vi "GetRxPower(LC).vi"(0 "SAVE FILE PATH":path=path "C:/RageATE/Automated Tests/Tetra WAM/DVT/rxdata.csv", 1 "CloseCOM4":bool, 2 "RXAnt":i32=1, 3 "RunAM_Init":bool=TRUE, 4 "UseFastData(T)":bool=TRUE, 5 "error in (no error)":errorcluster, 6 "dBFS Ofset":dbl, 7 "SAVE TO FILE(T)":bool, 8 "INPUT FILE PATH":path, 9 "INPUT FROM FILE(T)":bool, 11 "CF(MHZ)":dbl=10.0 min=0.0 max=150.0 format="%#_13g", 13 "BW(MHZ)":dbl=10.0 format="%#_13g", 15 "AMInitDyn(t)":bool, 18 "#ofAvg":i32=1) -> (10 "band (dbfs/mhz)":dbl[](array[numeric])=[-40.41732245857817, 9.96580361504641] format="%#_4g", 12 "peak (dbfs/mhz)":dbl[](array[numeric])=[-43.929, 10.039082] format="%#_8g", 14 "Locked?(T)":bool=TRUE, 16 "Am_Init_Flag":bool, 19 "error out":errorcluster={"status"=FALSE, "code"=1073676418, "source"="VISA Close in GetRxPower.vi"})   [LabVIEW 2018]
uses:
  Tetra_Globals.vi
  Initialize References/Sequence Globals.vi
panel:
  out "PyBase":string
  out "Navg":string
  out "Fs":string
  in  "ForceRevC(t)":bool
  out "vipath":string
  out "antenna":string
  out "match substring":string
  out "py_comport":string
  out "gui working directory":path=path "C:/TetraLabGUI"
  in  "Plot":u16(ring) items=["NoPlot", "Plot"]
  out "standard error":string
  out "UseAVG(t)":bool
  out "cmd_in":string
  out "standard output":string="2939 49c4\r\n403 6001\r\nFound COM4\r\nseq off\r\nwr reg 0x02 0x0400\r\nwr reg 0x03 0x0000\r\nwr reg 0x04 1032\r\nwr reg 0x05 4\r\nwr reg 0x06 10\r\nwr reg 0x08 256\r\nwr reg 0x09 51\r\nwr reg 0x0A 4\r\nwr reg 0x0E 8000\r\nwr reg 0x0F 0x5555\r\nwr reg 0x10 0x0055\r\nwr reg 0x11 0xAAAA\r\nwr reg 0x12 0x00AA\r\nwr reg 0x1A 0x0000\r\nwr reg 0x1B 0x0000\r\nwr reg 0x17 0x0300\r\nwr reg 0x18 0x0000\r\nsos\r\n"
  out "Time(ms)":u32=1465
  out "start":u32=9009331
  out "console  output":string="b'OK\\n\\r'\r\n[-26 -27 -23 ... -15 -16 -17]\r\nMax Value: -43.929 dBFS at 10.039082 MHz\r\nCF_OUT(MHz) = 9.96580361504641\r\nBP_OUT(dBfs) = -40.41732245857817\r\n"
  # "Input Dialog. Check \"Show Plot\" if desired"
  # "7.06"
  # "File Path Dialog. Check if file save desired"
  # "Band  & Peak Power Outputs"
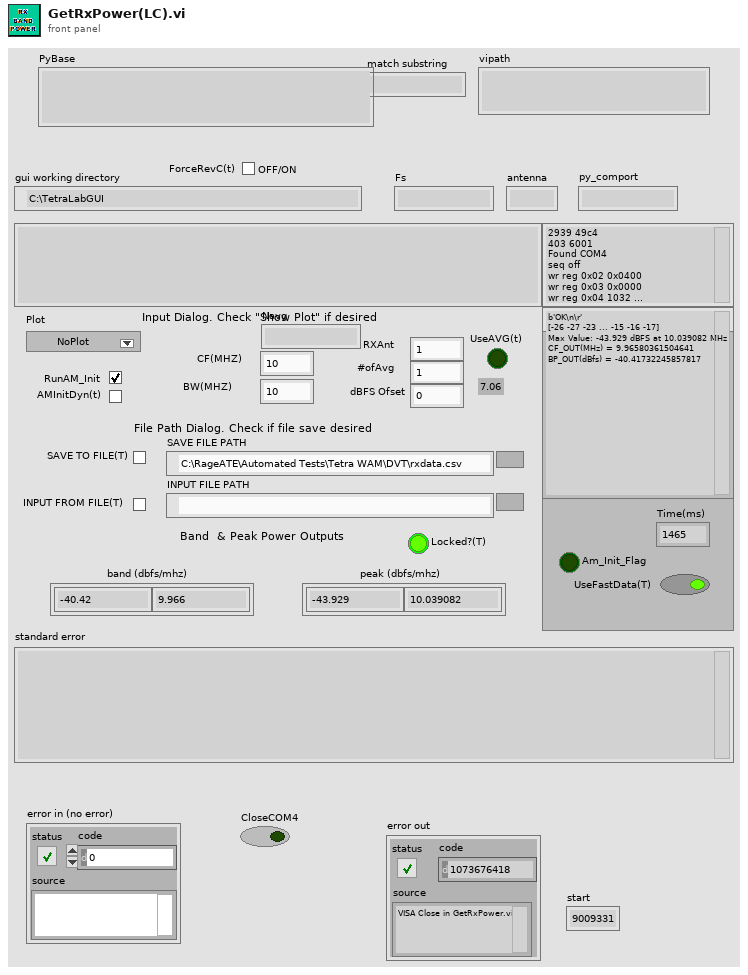
[diagram p1: front panel]
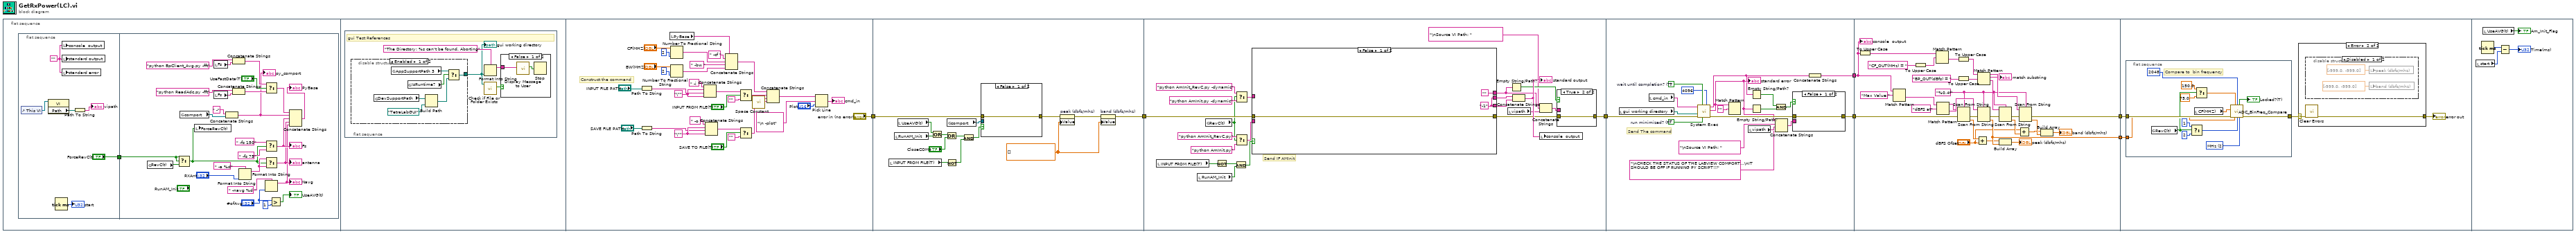
[diagram p0: block diagram]
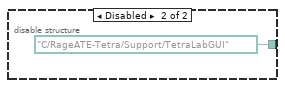
[diagram p2: hidden frame]
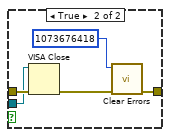
[diagram p4: hidden frame]
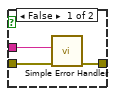
[diagram p5: hidden frame]
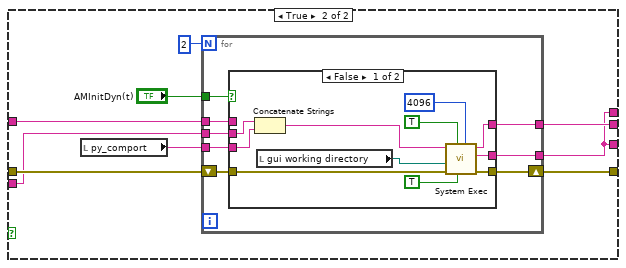
[diagram p6: hidden frame]
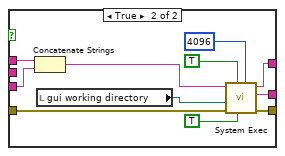
[diagram p7: hidden frame]
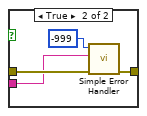
[diagram p8: hidden frame]
diagram:
  n1 = flat-sequence {
    tunnel: ["error in (no error)"] -> w1
    tunnel: [w100] -> w2
    tunnel: w1 -> [w99]
    tunnel: [w119] -> w5
    tunnel: w2 -> [w128]
    tunnel: [w189] -> w7
    tunnel: [w184] -> w6
    tunnel: w5 -> [w191]
    tunnel: w7 -> [w227]
    tunnel: w6 -> [w211]
    tunnel: [w212] -> w4
    tunnel: [w210] -> w3
    tunnel: w4 -> [w233]
    tunnel: w3 -> [w232]
    frame #0 {
      n2 = flat-sequence {
        tunnel: ["ForceRevC(t)"] -> w8
        tunnel: w8 -> [w35]
        frame #0 {
          w13 = ""
          n3 = control-ref of="This VI"() -> (w10:refnum<vi>)
          n4 = property class="VI"(reference=w10) -> ("Path"=w11:path)  [unwired: 1 in, 2 out]
          n5 = Tick Count (ms)() -> (millisecond timer value=→"start":u32)
          n6 = local write "console  output"(w13) -> ()
          n7 = local write "standard output"(w13) -> ()
          n8 = local write "standard error"(w13) -> ()
          n9 = Path To String(path=w11) -> (string=→"vipath":string)
        }
        frame #1 {
          n10 = global read "Tetra_Globals.vi" "RevC(t)"() -> (w36:bool)
          n11 = Select(t=w35, s=w35, f=w36) -> (s? t:f=w33:bool)
          n12 = global read "Tetra_Globals.vi" "comport"() -> (w39:refnum<visa-resource-name>)
          n13 = local write "ForceRevC(t)"(w33) -> ()
          n14 = local read "Fs"() -> (w26:string)
          n15 = local read "Fs"() -> (w27:string)
          n16 = Concatenate Strings(" -" ("string"), w39) -> (w19:string)
          "py_comport" <- w19
          n17 = Concatenate Strings("python BpClient_Avg.py -fft" ("command line"), w26) -> (w23:string)
          n18 = Concatenate Strings("python ReadAdc.py -fft" ("command line"), w27) -> (w22:string)
          n19 = Format Into String(format string=" -a %d", "RXAnt") -> (resulting string=w37:string)  [unwired: 2 in, 1 out]
          n20 = Select(t=w23, s="UseFastData(T)", f=w22) -> (s? t:f=w20:string)
          n21 = Select(t=" -fs 150" ("format string"), s=w33, f=" -fs 75" ("format string")) -> (s? t:f=w18:string)
          "Fs" <- w18
          n22 = Select(t=w37, s=w33, f=w37) -> (s? t:f=w17:string)
          "antenna" <- w17
          n23 = Format Into String(format string=" -navg %d " ("string"), "#ofAvg") -> (resulting string=w16:string)  [unwired: 2 in, 1 out]
          "Navg" <- w16
          n24 = Greater?(x="#ofAvg", y=1 ("x")) -> (0:→"UseAVG(t)":bool)
          n25 = Concatenate Strings(w20, w19, w18, w17, w16) -> (→"PyBase":string)
        }
      }
    }
    frame #1 {
      n26 = flat-sequence {
        frame #0 {
          # "gui Test References"
          n27 = disable-structure shown="Enabled" {
            disable-tunnel: [w46 path "C:/RageATE-Tetra/Support/TetraLabGUI" ("path")] -> w43
            frame Enabled {
              n28 = global read "Sequence Globals.vi" "DevSupportPath"() -> (w49:path)
              n29 = global read "Sequence Globals.vi" "AppSupportPath 3"() -> (w50:path)
              n30 = global read "Sequence Globals.vi" "IsRuntime?"() -> (w51:bool)
              n31 = Build Path(base path=w49, name or relative path=path "TetraLabGUI" ("gui working directory")) -> (appended path=w47:path)
              n32 = Select(t=w50, s=w51, f=w47) -> (s? t:f=w46:path)
            }
            frame Disabled {
            }
          }
          "gui working directory" <- w43
          n33 = Format Into String(format string="The Directory: %s can't be found. Aborting", w43) -> (resulting string=w42:string)  [unwired: 2 in, 1 out]
          n34 = call <vilib>:"Check if File or Folder Exists.vi"("path"=w43) -> ("file or folder exists?"=w45:bool)  [unwired: 8 in, 2 out]
          n35 = case shown="False" w45 {
            tunnel: w42 -> [w53 _]
            frame False {
              n36 = call "Display Message to User"("Message"=w53) -> ("OK"=w54:bool)  [unwired: 9 in, 1 out]
              n37 = Stop(stop? (T)=w54) -> ()
            }
            frame True {
            }
          }
        }
      }
    }
    frame #2 {
      w62 = "\"" ("string")
      w71 = "\"" ("string")
      # "Construct the command"
      n38 = Path To String(path="INPUT FILE PATH") -> (string=w65:string)
      n39 = Path To String(path="SAVE FILE PATH") -> (string=w69:string)
      n40 = local read "PyBase"() -> (w55:string)
      n41 = Number To Fractional String(number="CF(MHZ)", precision (6)=i16 2) -> (F-format string=w84:string)  [unwired: 2 in]
      n42 = Number To Fractional String(number="BW(MHZ)", precision (6)=i16 2) -> (F-format string=w85:string)  [unwired: 2 in]
      n43 = Concatenate Strings(" -i " ("string"), w62, w65, w62) -> (w60:string)
      n44 = Concatenate Strings(" -o " ("string"), w71, w69, w71) -> (w68:string)
      n45 = Concatenate Strings(w55, " -cf " ("string"), w84, " -bw " ("string"), w85) -> (w86:string)
      n46 = Select(t=w60, s="INPUT FROM FILE(T)", f="") -> (s? t:f=w59:string)
      n47 = Select(t=w68, s="SAVE TO FILE(T)", f="") -> (s? t:f=w58:string)
      n48 = call <vilib>:"Space Constant.vi"() -> ("String"=w73:string)
      n49 = Concatenate Strings(w86, w59, w58, w73) -> (w74:string)
      n50 = Pick Line(string ("")=w74, multi-line string="\n -plot", line index="Plot") -> (output string=→"cmd_in":string)
    }
    frame #3 {
      w97 = dbl[] [] ("peak (dbfs/mhz)")
      n51 = local read "INPUT FROM FILE(T)"() -> (w88:bool)
      n52 = local read "RunAM_Init"() -> (w94:bool)
      n53 = local read "UseAVG(t)"() -> (w92:bool)
      n54 = Or(x=w92, y=w94) -> (x .or. y?=w95:bool)
      n55 = Or(x=w95, y="CloseCOM4") -> (x .or. y?=w89:bool)
      n56 = Not(x=w88) -> (.not. x?=w87:bool)
      n57 = global read "Tetra_Globals.vi" "comport"() -> (w91:refnum<visa-resource-name>)
      n58 = And(x=w89, y=w87) -> (x .and. y?=w90:bool)
      n59 = case shown="False" w90 {
        tunnel: w99 -> [w101 w106]
        tunnel: [w101 w103] -> w96
        tunnel: w91 -> [_ w102]
        frame False {
        }
        frame True {
          n60 = VISA Close(VISA resource name=w102, error in (no error)=w106) -> (error out=w104:errorcluster)
          n61 = call <vilib>:"Clear Errors.vi"("error in (no error)"=w104, "specific error code to clear (0: all)"=1073676418) -> ("error out"=w103:errorcluster)  [unwired: 4 in, 1 out]
        }
      }
      n62 = property on="peak (dbfs/mhz)" class="Arr (strict)"(error in=w96, "Value"=w97) -> (error out=w98:errorcluster)  [unwired: 1 in, 1 out]
      n63 = property on="band (dbfs/mhz)" class="Arr (strict)"(error in=w98, "Value"=w97) -> (error out=w100:errorcluster)  [unwired: 1 in, 1 out]
    }
    frame #4 {
      # "Send IF AMInit"
      n64 = local read "INPUT FROM FILE(T)"() -> (w122:bool)
      n65 = local read "RunAM_Init"() -> (w127:bool)
      n66 = global read "Tetra_Globals.vi" "RevC(t)"() -> (w107:bool)
      n67 = Not(x=w122) -> (.not. x?=w121:bool)
      n68 = And(x=w121, y=w127) -> (x .and. y?=w123:bool)
      n69 = Select(t="python AmInit_RevC.py -dynamic" ("command line"), s=w107, f="python AmInit.py -dynamic" ("command line")) -> (s? t:f=w108:string)
      n70 = Select(t="python AmInit_RevC.py" ("command line"), s=w107, f="python AmInit.py" ("command line")) -> (s? t:f=w109:string)
      n71 = case shown="False" w123 {
        tunnel: [w135 w144] -> w120
        tunnel: w128 -> [w135 w143]
        tunnel: [w134 w142] -> w126
        tunnel: [w134 w138] -> w125
        tunnel: ["" w138] -> w117
        tunnel: w109 -> [_ w137]
        tunnel: w108 -> [_ w136]
        frame False {
          w134 = "-1" ("standard output")
        }
        frame True {
          n72 = local read "py_comport"() -> (w139:string)
          n73 = for {
            N: 2 -> [_]
            tunnel: [w150] -> w142
            tunnel: "AMInitDyn(t)" -> [w149]
            shift-right: [w152] -> w144
            shift-left: w143 -> [w151]
            tunnel: w139 -> [w148]
            tunnel: [w147] -> w138
            tunnel: w137 -> [w146]
            tunnel: w136 -> [w145]
            n74 = case shown="False" w149 {
              tunnel: [w163 w174] -> w152
              tunnel: w151 -> [w160 w171]
              tunnel: [w159 w170] -> w150
              tunnel: w148 -> [w155 w166]
              tunnel: [w154 w165] -> w147
              tunnel: w146 -> [w153 _]
              tunnel: w145 -> [_ w164]
              frame False {
                n75 = Concatenate Strings(w153, w155) -> (w156:string)
                n76 = local read "gui working directory"() -> (w157:path)
                n77 = call <vilib>:"System Exec.vi"("expected output size  (4096)"=u32 4096, "run minimized? (F)"=TRUE, "wait until completion? (T)"=TRUE, "error in (no error)"=w160, "working directory"=w157, "command line"=w156) -> ("error out"=w163:errorcluster, "standard error"=w154:string, "standard output"=w159:string)  [unwired: 2 in, 1 out]
              }
              frame True {
                n78 = Concatenate Strings(w164, w166) -> (w167:string)
                n79 = local read "gui working directory"() -> (w168:path)
                n80 = call <vilib>:"System Exec.vi"("expected output size  (4096)"=u32 4096, "run minimized? (F)"=TRUE, "wait until completion? (T)"=TRUE, "error in (no error)"=w171, "working directory"=w168, "command line"=w167) -> ("error out"=w174:errorcluster, "standard error"=w165:string, "standard output"=w170:string)  [unwired: 2 in, 1 out]
              }
            }
          }
        }
      }
      n81 = local read "vipath"() -> (w115:string)
      n82 = Empty String/Path?(string/path=w117) -> (empty?=w118:bool)
      n83 = Concatenate Strings(w126, w125) -> (w124:string)
      "standard output" <- w124
      n84 = Concatenate Strings(w117, "\nSource VI Path: ", w115) -> (w116:string)
      n85 = local write "console  output"(w124) -> ()
      n86 = case shown="True" w118 {
        tunnel: w120 -> [w131 w132]
        tunnel: [w130 w132] -> w119
        tunnel: w116 -> [w129 _]
        frame False {
          n87 = call <vilib>:"Simple Error Handler.vi"("error source (\" \")"=w129, "error in (no error)"=w131) -> ("error out"=w130:errorcluster)  [unwired: 3 in, 4 out]
        }
        frame True {
        }
      }
    }
    frame #5 {
      w192 = TRUE  # wait until completion? (T)
      w193 = TRUE  # run minimized? (F)
      # "Send The command"
      n88 = local read "gui working directory"() -> (w187:path)
      n89 = local read "cmd_in"() -> (w188:string)
      n90 = call <vilib>:"System Exec.vi"("expected output size  (4096)"=u32 4096, "run minimized? (F)"=w193, "wait until completion? (T)"=w192, "error in (no error)"=w191, "working directory"=w187, "command line"=w188) -> ("error out"=w185:errorcluster, "standard error"=w180:string, "standard output"=w175:string)  [unwired: 2 in, 1 out]
      "standard error" <- w180
      n91 = Match Pattern(string=w180, regular expression="") -> ()  [unwired: 1 in, 4 out]
      n92 = local read "vipath"() -> (w181:string)
      n93 = Empty String/Path?(string/path=w175) -> (empty?=w176:bool)
      n94 = Empty String/Path?(string/path=w180) -> (empty?=w183:bool)
      n95 = And(x=w176, y=w183) -> (x .and. y?=w177:bool)
      n96 = Concatenate Strings(w180, "\nSource VI Path: ", w181, "\nCHECK THE STATUS OF THE LABVIEW COMPORT...\nIT SHOULD BE OFF IF RUNNING PY SCRIPT!!!" ("string")) -> (w179:string)
      n97 = case shown="False" w177 {
        tunnel: w185 -> [w194 w197]
        tunnel: [w194 w196] -> w184
        tunnel: w179 -> [_ w195]
        frame False {
        }
        frame True {
          n98 = call <vilib>:"Simple Error Handler.vi"("error code (no error:0)"=-999, "error source (\" \")"=w195, "error in (no error)"=w197) -> ("error out"=w196:errorcluster)  [unwired: 2 in, 4 out]
        }
      }
      n99 = Concatenate Strings(w175) -> (w189:string)
    }
    frame #6 {
      w216 = "%0.4f" ("format string")
      n100 = To Upper Case(1:w227) -> (0:w199:string)
      n101 = Match Pattern(string=w227, regular expression="Max Value:") -> (after substring=w223:string)  [unwired: 1 in, 3 out]
      n102 = To Upper Case(1:"CF_OUT(MHz) = " ("regular expression")) -> (0:w200:string)
      n103 = Match Pattern(string=w199, regular expression=w200) -> (after substring=w219:string)  [unwired: 1 in, 3 out]
      n104 = Match Pattern(string=w223, regular expression="dBFS at") -> (before substring=w224:string, after substring=w225:string)  [unwired: 1 in, 2 out]
      n105 = To Upper Case(1:w219) -> (0:w202:string)
      n106 = To Upper Case(1:"BP_OUT(dBfs) = " ("regular expression")) -> (0:w201:string)
      n107 = Scan From String(format string=w216, input string=w224, error in=w211) -> (error out=w209:errorcluster, output 1=w228:dbl)  [unwired: 2 in, 2 out]
      n108 = Add(x=w228, y="dBFS Ofset") -> (x+y=w206:dbl)
      n109 = Match Pattern(string=w202, regular expression=w201) -> (before substring=w218:string, match substring=→"match substring":string, after substring=w217:string)  [unwired: 1 in, 1 out]
      n110 = Scan From String(format string=w216, input string=w225, error in=w209) -> (error out=w208:errorcluster, output 1=w212:dbl)  [unwired: 2 in, 2 out]
      n111 = Scan From String(format string=w216, input string=w217, error in=w208) -> (error out=w207:errorcluster, output 1=w214:dbl)  [unwired: 2 in, 2 out]
      n112 = Build Array(w206, w212) -> (→"peak (dbfs/mhz)":dbl[])
      n113 = Add(x="dBFS Ofset", y=w214) -> (x+y=w205:dbl)
      n114 = Scan From String(format string=w216, input string=w218, error in=w207) -> (error out=w210:errorcluster, output 1=w213:dbl)  [unwired: 2 in, 2 out]
      n115 = Build Array(w205, w213) -> (→"band (dbfs/mhz)":dbl[])
      "console  output" <- w227
    }
    frame #7 {
      n116 = flat-sequence {
        tunnel: [w251] -> w231
        tunnel: w232 -> [w248]
        tunnel: w233 -> [w247]
        frame #0 {
          w249 = u16 2 items=["Hz", "KHz", "MHz"] ("F units")
          # "Compare to  bin frequency"
          n117 = global read "Tetra_Globals.vi" "RevC(t)"() -> (w239:bool)
          n118 = Select(t=1 ("+/- error(bins)"), s=w239, f=2 ("+/- error(bins)")) -> (s? t:f=w243:i32)
          n119 = local read "CF(MHZ)"() -> (w246:dbl)
          n120 = Select(t=150.0 ("Fs(MHZ)"), s=w239, f=75.0 ("Fs(MHZ)")) -> (s? t:f=w245:dbl)
          n121 = call "ADC_BinFreq_Compare.vi"("Fsample"=w245, "# of Samples"=2048, "Expected Frequency"=w246, "error in"=w248, "Input Freq"=w247, "+/- error(bins)"=w243, "F units"=w249) -> ("In Range?(T)"=→"Locked?(T)":bool, "error out"=w251:errorcluster)  [unwired: 5 in, 2 out]
        }
      }
      n122 = case shown="Error" w231 {
        selector: w231 -> [w234 w236]
        tunnel: [w234 w235] -> w230
        frame No Error {
        }
        frame Error {
          n123 = disable-structure shown="Disabled" {
            frame Disabled {
              n124 = local write "peak (dbfs/mhz)"(dbl[] [-999.0, -999.0] ("peak (dbfs/mhz)")) -> ()
              n125 = local write "band (dbfs/mhz)"(dbl[] [-999.0, -999.0] ("band (dbfs/mhz)")) -> ()
            }
            frame Enabled {
            }
          }
          n126 = call <vilib>:"Clear Errors.vi"("error in (no error)"=w236) -> ("error out"=w235:errorcluster)  [unwired: 5 in, 1 out]
        }
      }
      "error out" <- w230
    }
    frame #8 {
      n127 = local read "start"() -> (w255:u32)
      n128 = Tick Count (ms)() -> (millisecond timer value=w256:u32)
      n129 = local read "UseAVG(t)"() -> (→"Am_Init_Flag":bool)
      n130 = Subtract(x=w256, y=w255) -> (x-y=→"Time(ms)":u32)
    }
  }
